vi "Dashboard Main.vi"() -> ()   [LabVIEW 2018]
uses:
  <vilib>/Utility/miscctls.llb/LVRowAndColumnTypeDef.ctl
  <vilib>/event_ctls.llb/eventvkey.ctl
  <vilib>/Rock Robotics/Network Tables/NT Read Numeric Array.vi
  <vilib>/Rock Robotics/Network Tables/NT Write Boolean.vi
  <vilib>/Rock Robotics/Network Tables/NT Read Boolean.vi
  <vilib>/Rock Robotics/WPI/Dashboard/WPI_DashboardLogging Global.vi
panel:
  in  "Camera Settings Right":T1={"Frame Rate"=30, "Compression"=30, "Size"=1, "DB Camera Config"=FALSE} {"Frame Rate" scale=1.0..30.0; "Compression" scale=100.0..-1.0; "Size" items=["640x480", "320x240", "160x120"]}
  in  "Camera Name Right":string(combo)="No Camera Selection"
  out "Camera Perf":string
  in  "Camera Settings":T1={"Frame Rate"=30, "Compression"=30, "Size"=1, "DB Camera Config"=FALSE} {"Frame Rate" scale=1.0..30.0; "Compression" scale=100.0..-1.0; "Size" items=["640x480", "320x240", "160x120"]}
  in  "TCP":refnum<k5>
  in  "Rec Mode":enum32{"Stop", "Record", "Playback"}(radio)
  out "Robot IP":string
  out "Image Message":string="Timeout in Camera Communications"
  in  "Dashboard Tab":T2(tab)
  in  "Select Auto":string(combo)="Select Autonomous ..."
  out "NT Connection":bool
  out "MotorChart R":cluster{"Numeric":dbl, "Numeric":dbl}(graph)
  out "MotorChart L":cluster{"Numeric":dbl, "Numeric":dbl}(graph)
  out "MotorSliders R":cluster{"MotorSlide1":dbl, "MotorSlide2":dbl} {"MotorSlide2" scale=-1.0..1.0 scale format="%#_2e"; "MotorSlide1" scale=-1.0..1.0 scale format="%#_2e"}
  out "MotorSliders L":cluster{"MotorSlide1":dbl, "MotorSlide2":dbl} {"MotorSlide2" scale=-1.0..1.0 scale format="%#_2e"; "MotorSlide1" scale=-1.0..1.0 scale format="%#_2e"}
  out "Gyro":dbl(knob) scale=0.0..360.0
  out "JS1 Z":dbl(slide) scale=-1.0..1.0 scale format="%#_2e"
  out "JS1 Graph":cluster{"X":dbl, "Y":dbl}[](graph)
  out "JS1 Buttons":T3
  out "JS2 Z":dbl(slide) scale=-1.0..1.0 scale format="%#_2e"
  out "JS2 Graph":cluster{"X":dbl, "Y":dbl}[](graph)
  out "JS2 Buttons":T3
  out "Mode":T4(ring)=enum."Auto Disabled"
  out "Right Camera Perf":cluster{"Bandwidth (Mbps)":dbl, "FPS":dbl}
  out "Camera Image Right":T5(plugin-control)
  out "Right Drive Position":dbl
  out "Left Drive Position":dbl
  out "Right Drive Velocity":dbl
  out "Left Drive Velocity":dbl
  out "Hab 3 Triggered":bool
  out "Hatch Device Extended":bool
  out "Gyro 2":dbl(knob) scale=0.0..360.0
  out "Arm Orientation":string
  out "Arm Setpoint":string
  out "Elevator Setpoint":string
  in  "Part Two?":bool
  in  "Start Zone":string(combo)="1"
  in  "Start Position":string(combo)="left"
  in  "Autonomous Selection":string(combo)="0"
  in  "Test Slider":dbl(slide) scale=0.0..100.0 scale format="%#_3g"
  in  "On/Off":bool caption="Solenoid"
  in  "Test Name":u16(ring) items=["Select the test to run..."]
  in  "Test Tree":string(tree)
  in  "Motor":cluster{"Value":dbl, "Enable":bool} {"Value" scale=-1.0..1.0 scale format="%#_3g"}
  out "Progress":T6 {"Test Progress" scale=0.0..100.0}
  in  "Rev/Fwd":cluster{"Forward":bool, "Reverse":bool}
  in  "Test Ring":u16(ring) items=["Monochrome", "Color"]
  out "Cmd Status":string
  in  "Execute Command":bool
  in  "Command Params":string[][](table)
  in  "Command Selection":i32(listbox)
  in  "CheckList":i32(listbox)
  out "Tree":string(tree)
  out "Camera Image":T5(plugin-control)
  out "Background":bool
  in  "Camera Name":string(combo)="No Camera Selection"
  # "HW"
  # "HW"
  # "Joysticks"
  # "Drive Motors"
  # "Front"
  # "Left"
  # "Right"
  # "Back"
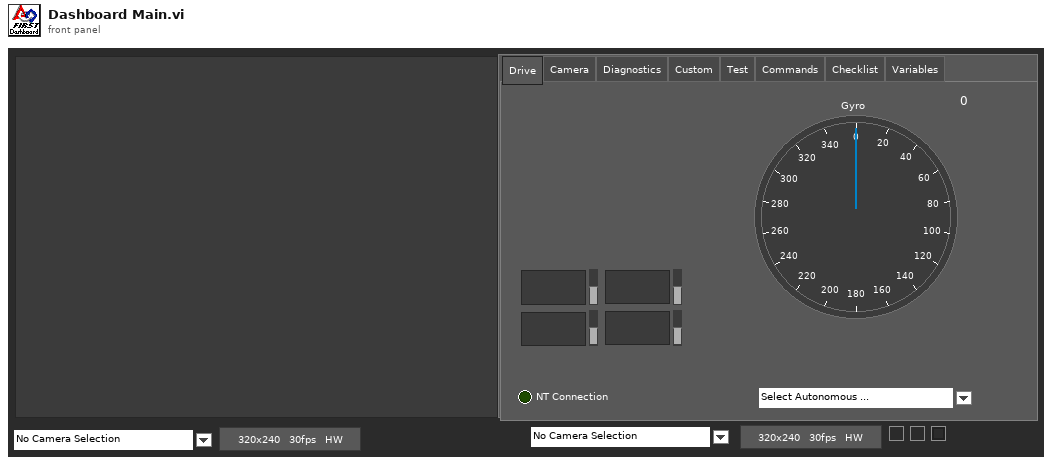
[diagram p1: front panel]
types:
  T1 = cluster{"Frame Rate":i32, "Compression":i32, "Size":u16, "DB Camera Config":bool}
  T2 = enum32{"Drive", "Camera", "Diagnostics", "Custom", "Test", "Commands", "Checklist", "Variables"}
  T3 = cluster{bool, bool, bool, bool, bool, bool, bool, bool, bool, bool, bool, bool}
  T4 = enum8{"Tele-Op Disabled", "Tele-Op Enabled", "Auto Disabled", "Auto Enabled", "Test Disabled", "Test Enabled", "Disconnected", "No Code", "E-Stop"}
  T5 = typedef "IMAQ Image.ctl" = refnum<image>
  T6 = cluster{"Test Progress":u8, "Test Progress Text":string}
  T7 = cluster{"Save Path":path, "Interval (s)":dbl, "Keep":i32}
  T8 = enum32{"Drive", "Camera", "Basic", "Custom", "Test", "Commands", "Checklist", "Variables"}
  T9 = typedef "Image Type" = u32
  T10 = cluster{"IDs":cluster{"RPC field ID":u16, "Unique ID":u16}, "String":string}
  T11 = cluster{"Error Strings":string, "Disable Counts":cluster{u16, u16}, "Rail Faults":cluster{u16, u16, u16}, "Robot IP":string, "DB Mode":u8, "Event Info":cluster{"Name":string, "Type":u8, "Number":u16, "Replay":u8}}
  T12 = cluster{"Storage":cluster{"Disk Free":u64, "RAM Block":u32, "RAM free":u32}, "CPU Utilization":cluster{"CPU % ISR":sgl, "CPU % Time Crit":sgl, "CPU % Timed Str":sgl, "CPU % High":sgl, "CPU % Above":sgl, "CPU % Normal":sgl, "CPU % Low":sgl}, "CAN":cluster{"% Bus Utilization":sgl, "Bus Off Cnt":u32, "TX_FIFO Full Cnt":u32, "Receive Error Cnt":u8, "Transmit Error Cnt":u8}, "HID":cluster{"HID Outputs":u32, "Rumble Low":u16, "Rumble High":u16}[]}
  T13 = cluster{"Status bits":cluster{"Test Mode":bool, "Autonomous":bool, "Enabled":bool, "Code Start":bool, "Brownout":bool, "Reserved 2":bool, "Reserved 3":bool, "E-Stop":bool}, "Code Trace":cluster{"Disabled":bool, "TeleOp":bool, "Auto":bool, "Test":bool}, "Controller Type":enum16{"unknown", "cRIO", "roboRio"}, "Code?":enum16{"unknown", "noCode", "code"}, "Battery V":dbl}
  T14 = cluster{"Control Bits":cluster{"TestMode":bool, "Autonomous":bool, "Enabled":bool, "FMS Present":bool, bool, bool, bool, "E-Stop":bool}, "Team Station ":u8, "Countdown":sgl, "Joystick Values":cluster{"Axes":dbl[], "Buttons":bool[], "POVs":i16[]}[]}
  T15 = cluster{"Axes":dbl[], "Buttons":bool[], "POVs":i16[]}[]
  T16 = cluster{"Axes":dbl[], "Buttons":bool[], "POVs":i16[]}
  T17 = cluster{"Buttons[0]":bool, "Buttons[1]":bool, "Buttons[2]":bool, "Buttons[3]":bool, "Buttons[4]":bool, "Buttons[5]":bool, "Buttons[6]":bool, "Buttons[7]":bool, "Buttons[8]":bool, "Buttons[9]":bool, "Buttons[10]":bool, "Buttons[11]":bool}
  T18 = cluster{"Camera Image":refnum<vi>, "Dashboard Tab":refnum<vi>, "Background":refnum<vi>, "Rec Mode":refnum<vi>, "Test Slider":refnum<vi>, "On/Off ":refnum<vi>, "Test Ring":refnum<vi>, "Rev/Fwd":refnum<vi>, "Test Name":refnum<vi>, "Motor":refnum<vi>, "Progress":refnum<vi>, "CheckList":refnum<vi>, "Tree":refnum<vi>, "Test Tree":refnum<vi>, "Command Params":refnum<vi>, "Command Selection":refnum<vi>, "Execute Command":refnum<vi>, "Cmd Status":refnum<vi>, "Camera Settings":refnum<vi>, "Camera Name":refnum<vi>, "Camera Perf":refnum<vi>, "Camera Settings Right":refnum<vi>, "Camera Name Right":refnum<vi>, "Camera Image Right":refnum<vi>}
  T19 = cluster{"Global Rectangle":i32[], "Contours":cluster{"Contour Type":u32, "ROI Type":u32, "Points":i32[]}[]}
  T20 = cluster{"Camera Name":string, string, "Saved DB Images Info":cluster{"Save Path":path, "Interval (s)":dbl, "Keep":i32}}
  T21 = cluster{"Camera Name Right":string, string, "Saved DB Images Info":cluster{"Save Path":path, "Interval (s)":dbl, "Keep":i32}}
  T22 = cluster{"Operation":enum16{"Update", "Clear"}, "Color Box":u32}[]
  T23 = typedef "eventvkey.ctl" = enum16{"ASCII", "Enter", "Return", "Shift", "Ctrl", "Alt", "Cmd", "Opt", "Caps", "NumLock", "Clear", "Break", "Up", "Down", "Left", "Right", "Insert", "Delete", "Home", "End", "PageUp", "PageDown", "Escape", "Help", "Pause", "ScrollLock", "F1", "F2", "F3", "F4", "F5", "F6", "F7", "F8", "F9", "F10", "F11", "F12", "F13", "F14", "F15", "F16", "F17", "F18", "F19", "F20", "F21", "F22", "F23", "F24", "Play", "VolumeUp", "VolumeDown", "Mute", "Two Byte Char"}
  T24 = cluster{"Image Size":bool, "Image Type":bool, "Pixel Value":bool, "ROI Information":bool, "Zoom Factor":bool}
  T25 = cluster{"Operation":enum16{"Update", "Clear"}, "Color Box":u32}
  T26 = typedef "LVRowAndColumnTypeDef.ctl" = cluster{"Row":i32, "Column":i32}
  T27 = cluster{"Shift":bool, "Ctrl":bool, "Alt":bool, "Cmd":bool, "Opt":bool}
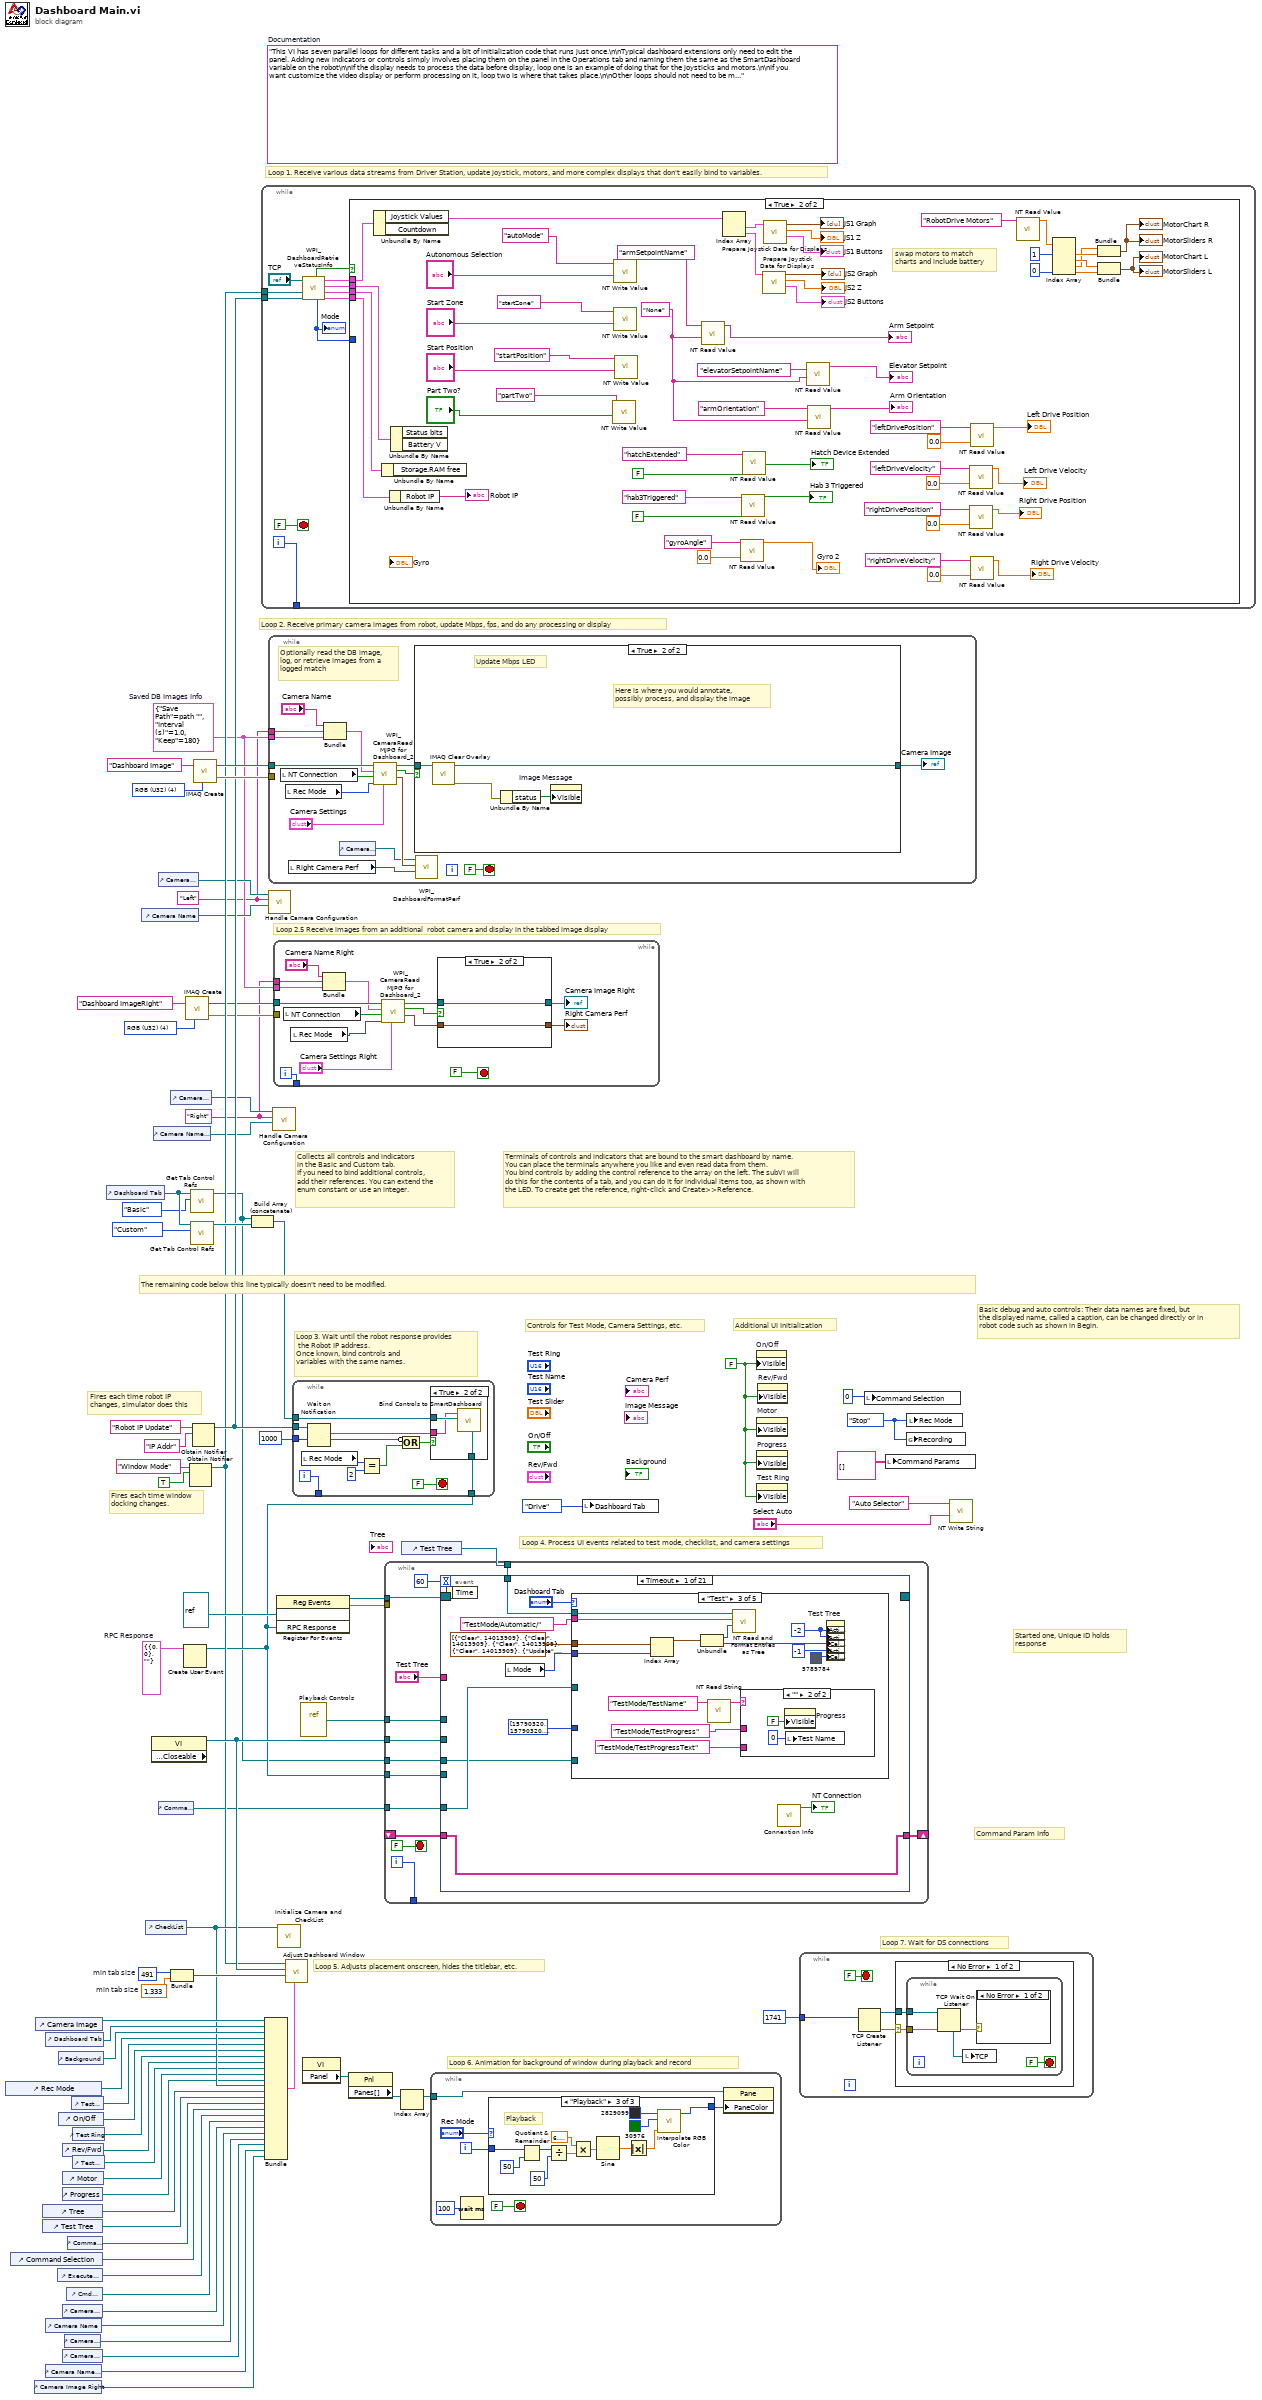
[diagram p0: block diagram]
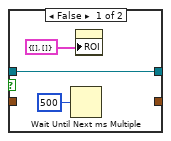
[diagram p2: hidden frame]
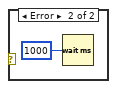
[diagram p3: hidden frame]
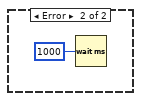
[diagram p4: hidden frame]
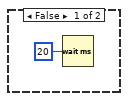
[diagram p5: hidden frame]
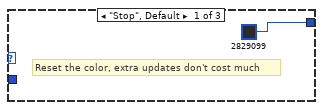
[diagram p6: hidden frame]
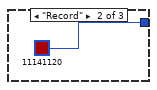
[diagram p7: hidden frame]
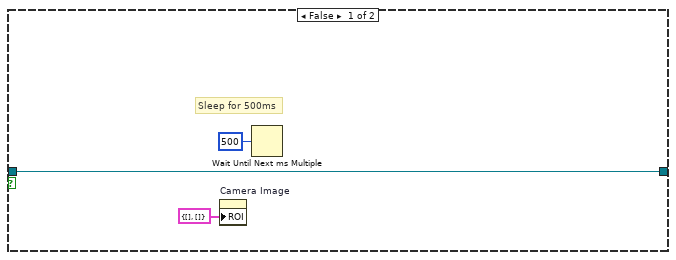
[diagram p9: hidden frame]
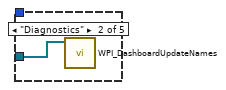
[diagram p11: hidden frame]
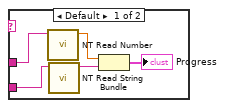
[diagram p12: hidden frame]
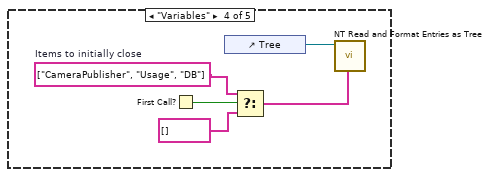
[diagram p13: hidden frame]
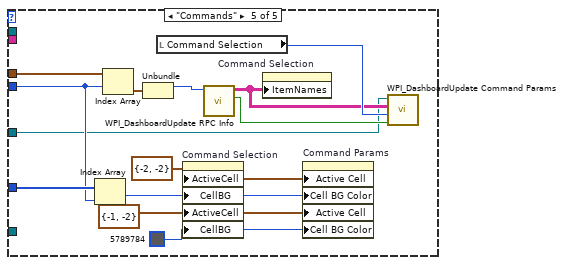
[diagram p14: hidden frame]
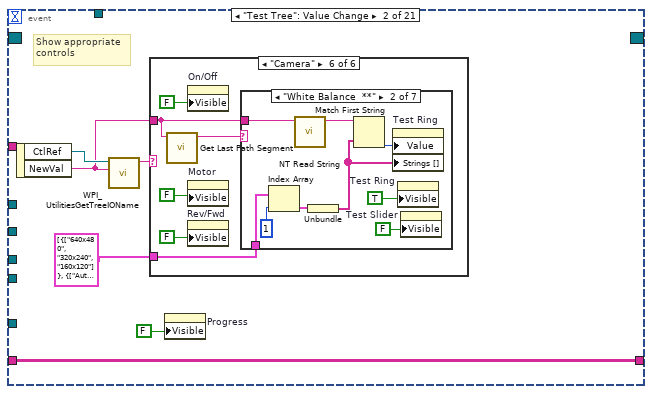
[diagram p15: hidden frame]
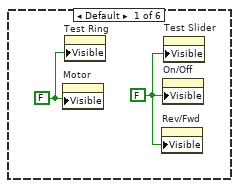
[diagram p16: hidden frame]
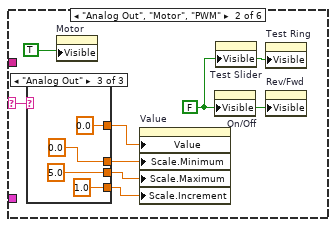
[diagram p17: hidden frame]
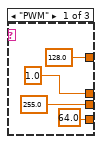
[diagram p18: hidden frame]
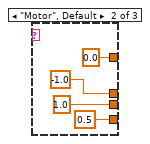
[diagram p19: hidden frame]
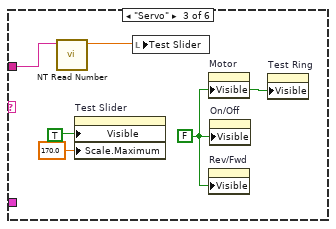
[diagram p20: hidden frame]
diagram:
  w4 = T7 {"Save Path"=path "", "Interval (s)"=1.0, "Keep"=180}  # Saved DB Images Info
  w3 = "Right"
  w2 = "Left"
  w14 = T9 4 items=["Grayscale (U8)", "Grayscale (I16)", "Grayscale (SGL)", "Complex (CSG)", "RGB (U32)", "HSL (U32)", "RGB (U64)"] ("Image Type")
  w30 = T10 {"IDs"={"RPC field ID"=0, "Unique ID"=0}, "String"=""}  # RPC Response
  w52 = 491  # min tab size
  w51 = 1.333  # min tab size
  w59 = enum32{"Stop", "Record", "Playback"}."Stop" ("Rec Mode")
  w36 = FALSE ("Visible")
  (unwired) "This VI has seven parallel loops for different tasks and a bit of initialization code that runs just once.\n\nTypical dashboard extensions only need to edit the panel. Adding new indicators or controls simply involves placing them on the panel in the Operations tab and naming them the same as the SmartDashboard variable on the robot\n\nIf the display needs to process the data before display, loop one is an example of doing that for the joysticks and motors.\n\nIf you want customize the video display or perform processing on it, loop two is where that takes place.\n\nOther loops should not need to be modified. They are pretty standard, and document the task they perform."  # Documentation
  w76 = T9 4 items=["Grayscale (U8)", "Grayscale (I16)", "Grayscale (SGL)", "Complex (CSG)", "RGB (U32)", "HSL (U32)", "RGB (U64)"] ("Image Type")
  # "Loop 2.5 Receive images from an additional  robot camera and display in the tabbed image display"
  # "Command Param Info"
  # "Started one, Unique ID holds\nresponse"
  # "Loop 7. Wait for DS connections"
  # "Basic debug and auto controls: Their data names are fixed, but\nthe displayed name, called a caption, can be changed directly or in\nrobot code such as shown in Begin."
  # "Controls for Test Mode, Camera Settings, etc."
  # "Additional UI Initialization"
  # "Loop 6. Animation for background of window during playback and record"
  # "Fires each time robot IP\nchanges, simulator does this"
  # "Fires each time window\ndocking changes."
  # "Collects all controls and indicators\nin the Basic and Custom tab.\nIf you need to bind additional controls,\nadd their references. You can extend the\nenum constant or use an integer."
  # "The remaining code below this line typically doesn't need to be modified."
  # "Loop 4. Process UI events related to test mode, checklist, and camera settings"
  # "Terminals of controls and indicators that are bound to the smart dashboard by name.\nYou can place the terminals anywhere you like and even read data from them.\nYou bind controls by adding the control reference to the array on the left. The subVI will\ndo this for the contents of a tab, and you can do it for individual items too, as shown with\nthe LED. To create get the reference, right-click and Create>>Reference."
  # "Loop 3. Wait until the robot response provides\n the Robot IP address.\nOnce known, bind controls and\nvariables with the same names."
  # "Loop 5. Adjusts placement onscreen, hides the titlebar, etc."
  # "Loop 1. Receive various data streams from Driver Station, update joystick, motors, and more complex displays that don't easily bind to variables."
  # "Loop 2. Receive primary camera images from robot, update Mbps, fps, and do any processing or display"
  n1 = control-ref of="Rec Mode"() -> (w42:refnum<vi>)
  n2 = control-ref of="Command Selection"() -> (w29:refnum<vi>)
  n3 = control-ref of="Camera Image Right"() -> (w7:refnum<vi>)
  n4 = control-ref of="Camera Image"() -> (w54:refnum<vi>)
  n5 = control-ref of="Tree"() -> (w46:refnum<vi>)
  n6 = control-ref of="Test Tree"() -> (w45:refnum<vi>)
  n7 = control-ref of="Dashboard Tab"() -> (w53:refnum<vi>)
  n8 = control-ref of="Camera Name"() -> (w20:refnum<vi>)
  n9 = control-ref of="Camera Name Right"() -> (w8:refnum<vi>)
  n10 = control-ref of="Execute Command"() -> (w31:refnum<vi>)
  n11 = control-ref of="Background"() -> (w49:refnum<vi>)
  n12 = control-ref of="On/Off"() -> (w40:refnum<vi>)
  n13 = control-ref of="Progress"() -> (w37:refnum<vi>)
  n14 = control-ref of="Camera Settings"() -> (w21:refnum<vi>)
  n15 = control-ref of="Camera Settings Right"() -> (w9:refnum<vi>)
  n16 = control-ref of="Rev/Fwd"() -> (w38:refnum<vi>)
  n17 = control-ref of="Motor"() -> (w43:refnum<vi>)
  n18 = control-ref of="Camera Perf"() -> (w19:refnum<vi>)
  n19 = control-ref of="Cmd Status"() -> (w25:refnum<vi>)
  n20 = control-ref of="Command Params"() -> (w32:refnum<vi>)
  n21 = control-ref of="Test Slider"() -> (w41:refnum<vi>)
  n22 = control-ref of="Test Ring"() -> (w39:refnum<vi>)
  n23 = control-ref of="Test Name"() -> (w44:refnum<vi>)
  n24 = control-ref of="Dashboard Tab"() -> (w57:refnum<vi>)
  n25 = control-ref of="Camera Name"() -> (w22:refnum<vi>)
  n26 = control-ref of="CheckList"() -> (w47:refnum<vi>)
  n27 = property class="VI" props=["Front Panel.Closeable"]() -> (reference out=w58:refnum<vi>)  [unwired: 2 in, 2 out]
  n28 = control-ref of="Camera Name Right"() -> (w10:refnum<vi>)
  n29 = control-ref of="Camera Settings"() -> (w23:refnum<vi>)
  n30 = control-ref of="Command Params"() -> (w24:refnum<vi>)
  n31 = control-ref of="Camera Settings Right"() -> (w11:refnum<vi>)
  n32 = Bundle("min tab size"=w52, "min tab size"=w51) -> (w50:cluster{"min tab size":i32, "min tab size":dbl})  [unwired: 1 in]
  n33 = Create User Event(user event datatype=w30) -> (user event=w26:refnum<user-event>)  [unwired: 1 in, 1 out]
  n34 = call "IMAQ Create"("Image Name"="Dashboard ImageRight", "Image Type"=w14) -> ("New Image"=w13:T5, "error out"=w12:errorcluster)  [unwired: 2 in, 1 out]
  n35 = Obtain Notifier(name (unnamed)="Window Mode", notification data type=TRUE) -> (notifier out=w34:refnum<notifier>)  [unwired: 2 in, 2 out]
  n36 = call <vilib>:"Get Tab Control Refs.vi"("Page Index"=T8."Basic" ("Dashboard Tab"), "TabControl in"=w57) -> ("ControlsOnPage"=w18:refnum<vi>[])  [unwired: 9 in]
  n37 = call <vilib>:"Get Tab Control Refs.vi"("Page Index"=T8."Custom" ("Dashboard Tab"), "TabControl in"=w57) -> ("ControlsOnPage"=w56:refnum<vi>[])  [unwired: 9 in]
  n38 = Obtain Notifier(name (unnamed)="Robot IP Update", notification data type="IP Addr" ("name (unnamed)")) -> (notifier out=w35:refnum<notifier>)  [unwired: 2 in, 2 out]
  n39 = call "IMAQ Create"("Image Name"="Dashboard Image", "Image Type"=w76) -> ("New Image"=w74:T5, "error out"=w73:errorcluster)  [unwired: 2 in, 1 out]
  n40 = Build Array (concatenate)(w18, w56) -> (w55:refnum<vi>[])
  n41 = while {
    tunnel: [w86] -> _
    tunnel: w35 -> [w80]
    tunnel: w34 -> [w77]
    i -> [w86]
    stop <- FALSE stop-if-true
    n42 = call <vilib>:"WPI_DashboardRetrieveStatusInfo.vi"("Binding Refnum"=w80, "Window Mode Notifier"=w77, "TCP Cnx"="TCP") -> ("Power and Errors"=w81:T11, "Robot Metrics"=w84:T12, "Status Info"=w85:T13, "Control Info"=w82:T14, "Robot Mode"=w79:T4, "Process?"=w83:bool)  [unwired: 3 in]
    "Mode" <- w79
    n43 = case shown="True" w83 {
      tunnel: w85 -> [_ w148]
      tunnel: w84 -> [_ w147]
      tunnel: w82 -> [_ w146]
      tunnel: w81 -> [_ w145]
      tunnel: w79 -> [_ _]
      frame False {
        n44 = Wait (ms)(milliseconds to wait=u32 20) -> ()  [unwired: 1 out]
      }
      frame True {
        w110 = "None" ("Default Value")
        # "swap motors to match\ncharts and include battery"
        n45 = Unbundle By Name(w146) -> ("Joystick Values"=w136:T15)  [unwired: 1 out]
        n46 = Unbundle By Name(w147) -> ()  [unwired: 1 out]
        n47 = Unbundle By Name(w145) -> ("Robot IP"=→"Robot IP":string)
        n48 = Unbundle By Name(w148) -> ()  [unwired: 2 out]
        n49 = call-poly <vilib>:"NT Write Value.vi"("Boolean"="Part Two?", "Name"="partTwo") -> ()  [unwired: 9 in, 1 out]
        n50 = call-poly <vilib>:"NT Write Value.vi"("String"="Autonomous Selection", "Name"="autoMode") -> ()  [unwired: 9 in, 1 out]
        n51 = call-poly <vilib>:"NT Write Value.vi"("String"="Start Zone", "Name"="startZone") -> ()  [unwired: 9 in, 1 out]
        n52 = call-poly <vilib>:"NT Write Value.vi"("String"="Start Position", "Name"="startPosition") -> ()  [unwired: 9 in, 1 out]
        n53 = call-poly <vilib>:"NT Read Value.vi"("Default Value"=w110, "Name"="armSetpointName") -> ("String"=→"Arm Setpoint":string)  [unwired: 8 in, 1 out]
        n54 = Index Array(array=w136) -> (element #1=w135:T16, element #2=w131:T16)  [unwired: 2 in]
        n55 = call-poly <vilib>:"NT Read Value.vi"("Default Value"=0.0, "Name"="gyroAngle") -> ("Numeric"=→"Gyro 2":dbl)  [unwired: 8 in, 1 out]
        n56 = call-poly <vilib>:"NT Read Value.vi"("Default Value"=FALSE, "Name"="hab3Triggered") -> ("Boolean"=→"Hab 3 Triggered":bool)  [unwired: 8 in, 1 out]
        n57 = call-poly <vilib>:"NT Read Value.vi"("Default Value"=FALSE, "Name"="hatchExtended") -> ("Boolean"=→"Hatch Device Extended":bool)  [unwired: 8 in, 1 out]
        n58 = call "Prepare Joystick Data for Displays.vi"("Joystick Values"=w131) -> ("Buttons"=→"JS2 Buttons":T17, "Z Axis"=→"JS2 Z":dbl, "Cartesian Data"=→"JS2 Graph":cluster{"X axis":dbl, "X axis":dbl}[])  [unwired: 8 in]
        n59 = call "Prepare Joystick Data for Displays.vi"("Joystick Values"=w135) -> ("Buttons"=→"JS1 Buttons":T17, "Z Axis"=→"JS1 Z":dbl, "Cartesian Data"=→"JS1 Graph":cluster{"X axis":dbl, "X axis":dbl}[])  [unwired: 8 in]
        n60 = call-poly <vilib>:"NT Read Value.vi"("Default Value"=w110, "Name"="elevatorSetpointName") -> ("String"=→"Elevator Setpoint":string)  [unwired: 8 in, 1 out]
        n61 = call-poly <vilib>:"NT Read Value.vi"("Default Value"=w110, "Name"="armOrientation") -> ("String"=→"Arm Orientation":string)  [unwired: 8 in, 1 out]
        n62 = call-poly <vilib>:"NT Read Value.vi"("Default Value"=0.0, "Name"="leftDriveVelocity") -> ("Numeric"=→"Left Drive Velocity":dbl)  [unwired: 8 in, 1 out]
        n63 = call-poly <vilib>:"NT Read Value.vi"("Default Value"=0.0, "Name"="rightDrivePosition") -> ("Numeric"=→"Right Drive Position":dbl)  [unwired: 8 in, 1 out]
        n64 = call-poly <vilib>:"NT Read Value.vi"("Default Value"=0.0, "Name"="leftDrivePosition") -> ("Numeric"=→"Left Drive Position":dbl)  [unwired: 8 in, 1 out]
        n65 = call-poly <vilib>:"NT Read Value.vi"("Default Value"=0.0, "Name"="rightDriveVelocity") -> ("Numeric"=→"Right Drive Velocity":dbl)  [unwired: 8 in, 1 out]
        n66 = call-poly <vilib>:"NT Read Value.vi"("Name"="RobotDrive Motors") -> ("Numeric Array"=w126:dbl[])  [unwired: 9 in, 1 out]
        n67 = Index Array(array=w126, index #1=1, index #4=0) -> (element #1=w140:dbl, element #2=w141:dbl, element #3=w139:dbl, element #4=w144:dbl)  [unwired: 2 in]
        n68 = Bundle("Numeric"=w139, "Numeric"=w140) -> (→"MotorChart R" →"MotorSliders R":cluster{"Numeric":dbl, "Numeric":dbl})  [unwired: 1 in]
        n69 = Bundle("Numeric"=w141, "Numeric"=w144) -> (→"MotorChart L" →"MotorSliders L":cluster{"Numeric":dbl, "Numeric":dbl})  [unwired: 1 in]
      }
    }
  }
  n70 = Bundle("Camera Image"=w54, "Dashboard Tab"=w53, "Background"=w49, "Rec Mode"=w42, "Test Slider"=w41, "On/Off"=w40, "Test Ring"=w39, "Rev/Fwd"=w38, "Test Name"=w44, "Motor"=w43, "Progress"=w37, "CheckList"=w47, "Tree"=w46, "Test Tree"=w45, "Command Params"=w32, "Command Selection"=w29, "Execute Command"=w31, "Cmd Status"=w25, "Camera Settings"=w21, "Camera Name"=w20, "Camera Perf"=w19, "Camera Settings Right"=w9, "Camera Name Right"=w8, "Camera Image Right"=w7) -> (w48:T18)  [unwired: 1 in]
  n71 = call "Handle Camera Configuration.vi"("CameraNameRef"=w22, "Display Name"=w2, "ClusterRef"=w23) -> ()  [unwired: 9 in]
  n72 = while {
    tunnel: w74 -> [w162]
    tunnel: w73 -> [_]
    tunnel: w4 -> [w155]
    tunnel: w2 -> [w152]
    stop <- FALSE stop-if-true
    # "Optionally read the DB image,\nlog, or retrieve images from a\nlogged match"
    n73 = local read "NT Connection"() -> (w156:bool)
    n74 = local read "Rec Mode"() -> (w159:enum32{"Stop", "Record", "Playback"})
    n75 = local read "Right Camera Perf"() -> (w150:cluster{"Bandwidth (Mbps)":dbl, "FPS":dbl})
    n76 = Bundle("Camera Name"="Camera Name", w152, "Saved DB Images Info"=w155) -> (w154:T20)  [unwired: 1 in]
    n77 = control-ref of="Camera Perf"() -> (w149:refnum<vi>)
    n78 = call <vilib>:"WPI_CameraRead MJPG for Dashboard_2.vi"("Camera Settings"="Camera Settings", "Rec Mode"=w159, "NT Connection"=w156, "Capture Info"=w154, "Image in"=w162) -> ("perf info"=w151:cluster{"Bandwidth (Mbps)":dbl, "fps":dbl}, "Active"=w160:bool, "Image\\ out"=w161:T5)  [unwired: 4 in]
    n79 = case shown="True" w160 {
      tunnel: w161 -> [w165 w168]
      tunnel: [w165 w167] -> w157
      frame False {
        # "Sleep for 500ms"
        n80 = property on="Camera Image" class="ImageControl"("ROI"=T19 {"Global Rectangle"=[], "Contours"=[]}) -> ()  [unwired: 2 in, 2 out]
        n81 = Wait Until Next ms Multiple(millisecond multiple=u32 500) -> ()  [unwired: 1 out]
      }
      frame True {
        # "Here is where you would annotate,\npossibly process, and display the image"
        # "Update Mbps LED"
        n82 = call "IMAQ Clear Overlay"("Image"=w168) -> ("error out"=w169:errorcluster, "Image Out"=w167:T5)  [unwired: 2 in, 7 out]
        n83 = Unbundle By Name(w169) -> ("status"=w170:bool)
        n84 = property on="Image Message" class="Str"("Visible"=w170) -> ()  [unwired: 2 in, 2 out]
      }
    }
    "Camera Image" <- w157
    n85 = call <vilib>:"WPI_DashboardFormatPerf.vi"("Right Camera Perf"=w150, "Performance"=w151, "String in"=w149) -> ()  [unwired: 9 in]
  }
  n86 = call "Handle Camera Configuration.vi"("CameraNameRef"=w10, "Display Name"=w3, "ClusterRef"=w11) -> ()  [unwired: 9 in]
  n87 = while {
    tunnel: w13 -> [w185]
    tunnel: w12 -> [_]
    tunnel: [w180] -> _
    tunnel: w4 -> [w176]
    tunnel: w3 -> [w173]
    i -> [w180]
    stop <- FALSE stop-if-true
    n88 = local read "NT Connection"() -> (w177:bool)
    n89 = local read "Rec Mode"() -> (w184:enum32{"Stop", "Record", "Playback"})
    n90 = Bundle("Camera Name Right"="Camera Name Right", w173, "Saved DB Images Info"=w176) -> (w175:T21)  [unwired: 1 in]
    n91 = call <vilib>:"WPI_CameraRead MJPG for Dashboard_2.vi"("Camera Settings"="Camera Settings Right", "Rec Mode"=w184, "NT Connection"=w177, "Capture Info"=w175, "Image in"=w185) -> ("perf info"=w171:cluster{"Bandwidth (Mbps)":dbl, "fps":dbl}, "Active"=w179:bool, "Image\\ out"=w182:T5)  [unwired: 4 in]
    n92 = case shown="True" w179 {
      tunnel: w182 -> [w187 w190]
      tunnel: [w187 w190] -> w178
      tunnel: [_ w189] -> w172
      tunnel: w171 -> [_ w189]
      frame False {
        n93 = Wait Until Next ms Multiple(millisecond multiple=u32 500) -> ()  [unwired: 1 out]
        n94 = property on="Camera Image Right" class="ImageControl"("ROI"=T19 {"Global Rectangle"=[], "Contours"=[]}) -> ()  [unwired: 2 in, 2 out]
      }
      frame True {
      }
    }
    "Camera Image Right" <- w178
    "Right Camera Perf" <- w172
  }
  n95 = register-events(refnum<vi> refnum, w26) -> (reference out=w63:refnum<event-registration>, error out=w62:errorcluster)  [unwired: 2 in]
  n96 = call "Initialize Camera and CheckList.vi"("ListBox in"=w47) -> ()  [unwired: 11 in]
  n97 = call "Adjust Dashboard Window.vi"("Sizing Refnums"=w48, "Size Constraints"=w50, "VI"=w58, "WIn Mode"=w34) -> ()  [unwired: 8 in]
  n98 = while {
    tunnel: w55 -> [w202]
    tunnel: w35 -> [w200]
    tunnel: [w198] -> _
    tunnel: u32 1000 ("milliseconds to wait") -> [w197]
    tunnel: w26 -> [w191]
    i -> [w198]
    stop <- FALSE stop-if-true
    n99 = local read "Rec Mode"() -> (w193:enum32{"Stop", "Record", "Playback"})
    n100 = Wait on Notification(notifier=w200, timeout in ms (-1)=w197) -> (notification=w199:string, timed out?=w195:bool)  [unwired: 2 in, 2 out]
    n101 = Equal?(x=w193, y=u16 2 ("Rec Mode")) -> (x = y?=w194:bool)
    n102 = Compound Arithmetic op=OR(invert w195, w194) -> (w196:bool)
    n103 = case shown="True" w196 {
      tunnel: w202 -> [_ w205]
      tunnel: w199 -> [_ w204]
      tunnel: w191 -> [_ w203]
      frame False {
      }
      frame True {
        n104 = call <vilib>:"Bind Controls to SmartDashboard.vi"("RPC ref"=w203, "Bound Control Refs"=w205, "Server IP Address"=w204) -> ()  [unwired: 9 in]
      }
    }
  }
  n105 = vi-ref "Playback Controls.vi"() -> (w64:refnum<vi>)
  n106 = property class="VI"() -> ("Panel"=w66:refnum<vi>)  [unwired: 2 in, 2 out]
  n107 = property class="Pnl"(reference=w66) -> ("Panes[]"=w67:refnum<vi>[])  [unwired: 1 in, 2 out]
  n108 = Index Array(array=w67) -> (element=w65:refnum<vi>)  [unwired: 1 in]
  n109 = control-ref of="Test Tree"() -> (w68:refnum<vi>)
  n110 = while {
    tunnel: [w215] -> _
    tunnel: w68 -> [w214]
    tunnel: w64 -> [w213]
    tunnel: w63 -> [w212]
    tunnel: w62 -> [_]
    tunnel: w58 -> [w211]
    tunnel: w26 -> [w210]
    tunnel: w24 -> [w209]
    shift-right: [w208] -> _
    shift-left: _ -> [w207]
    tunnel: w18 -> [w206]
    i -> [w215]
    stop <- FALSE stop-if-true
    n111 = event shown="[0] Timeout" {
      selector: w212 -> [_ _ _ _ _ _ _ _ _ _ _ _ _ _ _ _ _ _ _ _ _]
      dyn-events: [_ _ _ _ _ _ _ _ _ _ _ _ _ _ _ _ w475 _ _ _ _] -> _
      timeout: u32 60 ("milliseconds to wait") -> [_ _ _ _ _ _ _ _ _ _ _ _ _ _ _ _ _ _ _ _ _]
      tunnel: w214 -> [w227 _ _ _ _ _ _ _ _ _ _ _ _ _ _ _ _ _ _ _ _]
      tunnel: "Test Tree" -> [_ _ _ _ _ _ _ _ _ _ _ w442 w450 w452 w456 w464 _ _ _ _ _]
      tunnel: w213 -> [_ _ _ _ _ _ _ _ _ _ _ _ _ _ _ _ w477 _ w495 _ _]
      tunnel: w211 -> [_ _ _ _ _ _ _ _ _ _ _ _ _ _ _ _ w473 _ _ _ _]
      tunnel: w210 -> [_ _ _ _ _ _ _ _ _ _ _ _ _ _ _ _ w471 _ _ _ _]
      tunnel: w209 -> [w222 _ _ _ _ _ w393 _ _ _ _ _ _ _ _ _ _ _ _ _ _]
      tunnel: [w221 w270 w372 w377 w386 w390 w391 w400 w410 w417 w429 w441 w448 w451 w455 w463 w470 w490 w492 w496 w509] -> w208
      tunnel: w207 -> [w221 w270 w372 w377 w386 w390 w391 _ _ w417 w429 w441 w448 w451 w455 w463 w470 w490 w492 w496 w509]
      tunnel: w206 -> [w219 _ _ _ _ _ _ _ _ _ _ _ _ _ _ _ _ _ _ _ _]
      event Timeout {
        n112 = event-data() -> ()  [unwired: 1 in, 1 out]
        n113 = local read "Mode"() -> (w224:T4)
        n114 = case shown="\"Test\"" "Dashboard Tab" {
          tunnel: w227 -> [_ _ w243 _ _]
          tunnel: "TestMode/Automatic/" ("Name Pattern") -> [_ _ w242 _ _]
          tunnel: T22 [{"Operation"=enum."Clear", "Color Box"=14013909}, {"Operation"=enum."Clear", "Color Box"=14013909}, {"Operation"=enum."Clear", "Color Box"=14013909}, {"Operation"=enum."Clear", "Color Box"=14013909}, {"Operation"=enum."Update", "Color Box"=14013909}, {"Operation"=enum."Update", "Color Box"=16777215}, {"Operation"=enum."Clear", "Color Box"=14013909}, {"Operation"=enum."Clear", "Color Box"=14013909}, {"Operation"=enum."Clear", "Color Box"=14013909}] -> [_ _ w235 _ w263]
          tunnel: w224 -> [_ _ w234 _ w262]
          tunnel: u32[] [15790320, 15790320, 15790320, 15790320, 16777215, 16777215, 15790320, 15790320, 15790320] -> [_ _ _ _ w268]
          tunnel: w222 -> [_ _ _ _ w256]
          tunnel: w219 -> [_ w229 _ _ _]
          frame "Custom", Default {
          }
          frame "Diagnostics" {
            n115 = call <vilib>:"WPI_DashboardUpdateNames.vi"("Controls on Tab"=w229) -> ()  [unwired: 11 in]
          }
          frame "Test" {
            w241 = -2 ("Active Item:Row Number")
            n116 = Index Array(array=w235, index=w234) -> (element=w236:T25)
            n117 = Unbundle(w236) -> ("Operation"=w237:enum16{"Update", "Clear"}, "Color Box"=w238:u32)
            n118 = call <vilib>:"NT Read String.vi"("Name"="TestMode/TestName") -> ("String"=w232:string)  [unwired: 9 in, 1 out]
            n119 = call <vilib>:"NT Read and Format Entries as Tree.vi"("Operation"=w237, "Name Pattern"=w242, "Tree Refnum"=w243) -> ()  [unwired: 7 in, 2 out]
            n120 = case shown="\"\"" w232 {
              tunnel: "TestMode/TestProgress" ("Name") -> [w245 _]
              tunnel: "TestMode/TestProgressText" ("Name") -> [w244 _]
              frame Default {
                n121 = call <vilib>:"NT Read Number.vi"("Name"=w245) -> ("Numeric"=w246:dbl)  [unwired: 9 in, 1 out]
                n122 = call <vilib>:"NT Read String.vi"("Name"=w244) -> ("String"=w247:string)  [unwired: 9 in, 1 out]
                n123 = Bundle("Numeric"=w246, "String"=w247) -> (→"Progress":cluster{"Numeric":dbl, "String":string})  [unwired: 1 in]
              }
              frame "" {
                n124 = property on="Progress" class="Clust (strict)"("Visible"=FALSE) -> ()  [unwired: 2 in, 2 out]
                n125 = local write "Test Name"(u16 0) -> ()
              }
            }
            n126 = property on="Test Tree" class="Tree (strict)"("Active Item Row Number"=w241, "ActiveColNum"=w241, "CellBG"=w238, "Active Item Row Number"=-1 ("Active Item:Row Number"), "CellBG"=u32 5789784 ("Color Box")) -> ()  [unwired: 2 in, 2 out]
          }
          frame "Variables" {
            w253 = string[] ["CameraPublisher", "Usage", "DB"]  # Items to initially close
            n127 = First Call?() -> (First Call?: T/F=w254:bool)
            n128 = control-ref of="Tree"() -> (w255:refnum<vi>)
            n129 = Select(t=w253, s=w254, f=string[] []) -> (s? t:f=w251:string[])
            n130 = call <vilib>:"NT Read and Format Entries as Tree.vi"("Tags to  Close"=w251, "Tree Refnum"=w255) -> ()  [unwired: 8 in, 2 out]
          }
          frame "Commands" {
            w264 = u32 5789784 ("Color Box")
            w265 = T26 {"Row"=-1, "Column"=-2} ("Active Cell:Active Cell")
            w267 = T26 {"Row"=-2, "Column"=-2} ("Active Cell:Active Cell")
            n131 = Index Array(array=w268, index=w262) -> (element=w266:u32)
            n132 = Index Array(array=w263, index=w262) -> (element=w261:T25)
            n133 = Unbundle(w261) -> ("Operation"=w260:enum16{"Update", "Clear"})  [unwired: 1 out]
            n134 = local read "Command Selection"() -> (w259:i32)
            n135 = property on="Command Selection" class="MCListbox (strict)"("ActiveCell"=w267, "CellBG"=w266, "ActiveCell"=w265, "CellBG"=w264) -> ()  [unwired: 2 in, 2 out]
            n136 = call <vilib>:"WPI_DashboardUpdate RPC Info.vi"("Operation"=w260) -> ("update"=w258:bool, "commands"=w257:string[][])  [unwired: 9 in]
            n137 = property on="Command Selection" class="MCListbox (strict)"("ItemNames"=w257) -> ()  [unwired: 2 in, 2 out]
            n138 = property on="Command Params" class="Tbl (strict)"("Active Cell"=w267, "Cell BG Color"=w266, "Active Cell"=w265, "Cell BG Color"=w264) -> ()  [unwired: 2 in, 2 out]
            n139 = call <vilib>:"WPI_DashboardUpdate Command Params.vi"("Update"=w258, "NewVal"=w259, "Commands"=w257, "Param Tbl"=w256) -> ()  [unwired: 7 in, 1 out]
          }
        }
        n140 = call <vilib>:"Connextion Info.vi"() -> ("Connected"=→"NT Connection":bool)  [unwired: 10 in, 1 out]
      }
      event "Test Tree": Value Change {
        # "Show appropriate\ncontrols"
        n141 = event-data() -> ("CtlRef"=w273:refnum<vi>, "NewVal"=w271:string)  [unwired: 1 in]
        n142 = call <vilib>:"WPI_UtilitiesGetTreeIOName.vi"("NewVal"=w271, "TreeControl in"=w273) -> ("I/O Name"=w274:string)  [unwired: 9 in]
        n143 = case shown="\"Camera\"" w274 {
          selector: w274 -> [_ w281 _ w303 w312 _]
          tunnel: w271 -> [_ _ w300 w302 _ w319]
          tunnel: cluster{string[]}[] [{["640x480", "320x240", "160x120"]}, {["Auto", "Fixed indoor", "Fixed outdoor 1", "Fixed outdoor 2", "Fixed fluorescent 1", "Fixed fluorescent 2", "Hold current"]}, {["Auto", "Flicker-free 50 Hz", "Flicker-free 60 Hz", "Hold current"]}, {["None", "Prioritize frame rate", "Prioritize image quality"]}, {["Monochrome", "Color"]}] -> [_ _ _ _ _ w318]
          frame Default {
            w276 = FALSE ("Visible")
            w275 = FALSE ("Visible")
            n144 = property on="Motor" class="Clust (strict)"("Visible"=w275) -> ()  [unwired: 2 in, 2 out]
            n145 = property on="Test Ring" class="Ring (strict)"("Visible"=w275) -> ()  [unwired: 2 in, 2 out]
            n146 = property on="Rev/Fwd" class="Clust (strict)"("Visible"=w276) -> ()  [unwired: 2 in, 2 out]
            n147 = property on="On/Off" class="Bool (strict)"("Visible"=w276) -> ()  [unwired: 2 in, 2 out]
            n148 = property on="Test Slider" class="Slide (strict)"("Visible"=w276) -> ()  [unwired: 2 in, 2 out]
          }
          frame "Analog Out", "Motor", "PWM" {
            w282 = FALSE ("Visible")
            n149 = case shown="\"Analog Out\"" w281 {
              tunnel: [1.0 ("Value") -1.0 ("Value") 0.0 ("Value")] -> w280
              tunnel: [255.0 ("Value") 1.0 ("Value") 5.0 ("Value")] -> w279
              tunnel: [128.0 ("Value") 0.0 ("Value") 0.0 ("Value")] -> w278
              tunnel: [64.0 ("Value") 0.5 ("Value") 1.0 ("Value")] -> w277
              frame "PWM" {
              }
              frame "Motor", Default {
              }
              frame "Analog Out" {
              }
            }
            n150 = property on="Motor" class="Clust (strict)"("Visible"=TRUE) -> ()  [unwired: 2 in, 2 out]
            n151 = property on="Value" class="Slide (strict)"("Value"=w278, "Scale.Minimum"=w280, "Scale.Maximum"=w279, "Scale.Increment"=w277) -> ()  [unwired: 2 in, 2 out]
            n152 = property on="On/Off" class="Bool (strict)"("Visible"=w282) -> ()  [unwired: 2 in, 2 out]
            n153 = property on="Test Slider" class="Slide (strict)"("Visible"=w282) -> ()  [unwired: 2 in, 2 out]
            n154 = property on="Test Ring" class="Ring (strict)"("Visible"=w282) -> ()  [unwired: 2 in, 2 out]
            n155 = property on="Rev/Fwd" class="Clust (strict)"("Visible"=w282) -> ()  [unwired: 2 in, 2 out]
          }
          frame "Servo" {
            w298 = FALSE ("Visible")
            n156 = call <vilib>:"NT Read Number.vi"("Name"=w300) -> ("Numeric"=w299:dbl)  [unwired: 9 in, 1 out]
            n157 = property on="Test Slider" class="Slide (strict)"("Visible"=TRUE, "Scale.Maximum"=170.0 ("Scale.Range:Maximum")) -> ()  [unwired: 2 in, 2 out]
            n158 = local write "Test Slider"(w299) -> ()
            n159 = property on="Motor" class="Clust (strict)"("Visible"=w298) -> ()  [unwired: 2 in, 2 out]
            n160 = property on="Rev/Fwd" class="Clust (strict)"("Visible"=w298) -> ()  [unwired: 2 in, 2 out]
            n161 = property on="On/Off" class="Bool (strict)"("Visible"=w298) -> ()  [unwired: 2 in, 2 out]
            n162 = property on="Test Ring" class="Ring (strict)"("Visible"=w298) -> ()  [unwired: 2 in, 2 out]
          }
          frame "Relay", "Solenoid" {
            w301 = FALSE ("Visible")
            n163 = property on="Motor" class="Clust (strict)"("Visible"=w301) -> ()  [unwired: 2 in, 2 out]
            n164 = property on="Test Slider" class="Slide (strict)"("Visible"=w301) -> ()  [unwired: 2 in, 2 out]
            n165 = Search and Replace String(input string=w302, search string="/Value  **", replace string="/Direction") -> (result string=w308:string)  [unwired: 5 in, 3 out]
            n166 = property on="Test Ring" class="Ring (strict)"("Visible"=w301) -> ()  [unwired: 2 in, 2 out]
            n167 = call <vilib>:"NT Read String.vi"("Name"=w308) -> ("String"=w306:string)  [unwired: 9 in, 1 out]
            n168 = Equal?(x="Both directions", y=w306) -> (x = y?=w304:bool)
            n169 = Not(x=w304) -> (.not. x?=w305:bool)
            n170 = property on="Rev/Fwd" class="Clust (strict)"("Visible"=w304) -> ()  [unwired: 2 in, 2 out]
            n171 = property on="On/Off" class="Bool (strict)"("Visible"=w305, "Caption.Text"=w303) -> ()  [unwired: 2 in, 2 out]
          }
          frame "Compressor", "Digital Out" {
            w311 = FALSE ("Visible")
            # "Get direction and finish"
            n172 = property on="Motor" class="Clust (strict)"("Visible"=w311) -> ()  [unwired: 2 in, 2 out]
            n173 = property on="Test Slider" class="Slide (strict)"("Visible"=w311) -> ()  [unwired: 2 in, 2 out]
            n174 = property on="Test Ring" class="Ring (strict)"("Visible"=w311) -> ()  [unwired: 2 in, 2 out]
            n175 = property on="On/Off" class="Bool (strict)"("Visible"=TRUE, "Caption.Text"=w312) -> ()  [unwired: 2 in, 2 out]
            n176 = property on="Rev/Fwd" class="Clust (strict)"("Visible"=FALSE) -> ()  [unwired: 2 in, 2 out]
          }
          frame "Camera" {
            n177 = call <vilib>:"Get Last Path Segment.vi"("String in"=w319) -> ("String out"=w320:string)  [unwired: 10 in]
            n178 = property on="On/Off" class="Bool (strict)"("Visible"=FALSE) -> ()  [unwired: 2 in, 2 out]
            n179 = property on="Motor" class="Clust (strict)"("Visible"=FALSE) -> ()  [unwired: 2 in, 2 out]
            n180 = property on="Rev/Fwd" class="Clust (strict)"("Visible"=FALSE) -> ()  [unwired: 2 in, 2 out]
            n181 = case shown="\"White Balance  **\"" w320 {
              tunnel: w319 -> [w326 w335 w344 w353 w362 _ w368]
              tunnel: w318 -> [w324 w332 w341 w350 w359 _ _]
              frame "Size  **" {
                n182 = Index Array(array=w324) -> (element=w323:cluster{string[]})  [unwired: 1 in]
                n183 = call <vilib>:"NT Read String.vi"("Name"=w326) -> ("String"=w325:string)  [unwired: 9 in, 1 out]
                n184 = Unbundle(w323) -> (w321:string[])
                n185 = Match First String(2:w321, 3:w325) -> (0:w322:i32)  [unwired: 1 out]
                n186 = property on="Test Ring" class="Ring (strict)"("Value"=w322, "Strings []"=w321) -> ()  [unwired: 2 in, 2 out]
                n187 = property on="Test Ring" class="Ring (strict)"("Visible"=TRUE) -> ()  [unwired: 2 in, 2 out]
                n188 = property on="Test Slider" class="Slide (strict)"("Visible"=FALSE) -> ()  [unwired: 2 in, 2 out]
              }
              frame "White Balance  **" {
                n189 = Index Array(array=w332, index=1) -> (element=w333:cluster{string[]})
                n190 = call <vilib>:"NT Read String.vi"("Name"=w335) -> ("String"=w334:string)  [unwired: 9 in, 1 out]
                n191 = Unbundle(w333) -> (w330:string[])
                n192 = Match First String(2:w330, 3:w334) -> (0:w329:i32)  [unwired: 1 out]
                n193 = property on="Test Ring" class="Ring (strict)"("Value"=w329, "Strings []"=w330) -> ()  [unwired: 2 in, 2 out]
                n194 = property on="Test Ring" class="Ring (strict)"("Visible"=TRUE) -> ()  [unwired: 2 in, 2 out]
                n195 = property on="Test Slider" class="Slide (strict)"("Visible"=FALSE) -> ()  [unwired: 2 in, 2 out]
              }
              frame "Exposure  **" {
                n196 = Index Array(array=w341, index=2) -> (element=w342:cluster{string[]})
                n197 = call <vilib>:"NT Read String.vi"("Name"=w344) -> ("String"=w343:string)  [unwired: 9 in, 1 out]
                n198 = Unbundle(w342) -> (w338:string[])
                n199 = Match First String(2:w338, 3:w343) -> (0:w339:i32)  [unwired: 1 out]
                n200 = property on="Test Ring" class="Ring (strict)"("Value"=w339, "Strings []"=w338) -> ()  [unwired: 2 in, 2 out]
                n201 = property on="Test Ring" class="Ring (strict)"("Visible"=TRUE) -> ()  [unwired: 2 in, 2 out]
                n202 = property on="Test Slider" class="Slide (strict)"("Visible"=FALSE) -> ()  [unwired: 2 in, 2 out]
              }
              frame "Exposure Priority  **" {
                n203 = Index Array(array=w350, index=3) -> (element=w351:cluster{string[]})
                n204 = call <vilib>:"NT Read String.vi"("Name"=w353) -> ("String"=w352:string)  [unwired: 9 in, 1 out]
                n205 = Unbundle(w351) -> (w347:string[])
                n206 = Match First String(2:w347, 3:w352) -> (0:w348:i32)  [unwired: 1 out]
                n207 = property on="Test Ring" class="Ring (strict)"("Value"=w348, "Strings []"=w347) -> ()  [unwired: 2 in, 2 out]
                n208 = property on="Test Ring" class="Ring (strict)"("Visible"=TRUE) -> ()  [unwired: 2 in, 2 out]
                n209 = property on="Test Slider" class="Slide (strict)"("Visible"=FALSE) -> ()  [unwired: 2 in, 2 out]
              }
              frame "Color Enable  **" {
                n210 = Index Array(array=w359, index=4) -> (element=w360:cluster{string[]})
                n211 = call <vilib>:"NT Read String.vi"("Name"=w362) -> ("String"=w361:string)  [unwired: 9 in, 1 out]
                n212 = Unbundle(w360) -> (w356:string[])
                n213 = Match First String(2:w356, 3:w361) -> (0:w357:i32)  [unwired: 1 out]
                n214 = property on="Test Ring" class="Ring (strict)"("Value"=w357, "Strings []"=w356) -> ()  [unwired: 2 in, 2 out]
                n215 = property on="Test Ring" class="Ring (strict)"("Visible"=TRUE) -> ()  [unwired: 2 in, 2 out]
                n216 = property on="Test Slider" class="Slide (strict)"("Visible"=FALSE) -> ()  [unwired: 2 in, 2 out]
              }
              frame Default {
                n217 = property on="Test Ring" class="Ring (strict)"("Visible"=FALSE) -> ()  [unwired: 2 in, 2 out]
                n218 = property on="Test Slider" class="Slide (strict)"("Visible"=FALSE) -> ()  [unwired: 2 in, 2 out]
              }
              frame "Brightness  **", "Color Level  **", "Compression  **", "FPS  **", "Sharpness  **" {
                n219 = call <vilib>:"NT Read Number.vi"("Name"=w368) -> ("Numeric"=w367:dbl)  [unwired: 9 in, 1 out]
                n220 = local write "Test Slider"(w367) -> ()
                n221 = property on="Test Slider" class="Slide (strict)"("Visible"=TRUE, "Scale.Maximum"=100.0 ("Scale.Range:Maximum")) -> ()  [unwired: 2 in, 2 out]
                n222 = property on="Test Ring" class="Ring (strict)"("Visible"=FALSE) -> ()  [unwired: 2 in, 2 out]
              }
            }
          }
        }
        n223 = property on="Progress" class="Clust (strict)"("Visible"=FALSE) -> ()  [unwired: 2 in, 2 out]
      }
      event "Test Name": Mouse Enter {
        # "Populate the ring with the list of tests"
        n224 = event-data() -> ()  [unwired: 1 in, 1 out]
        n225 = call <vilib>:"NT Read String Array.vi"("Name"="TestMode/TestList") -> ("String Array"=w376:string[])  [unwired: 9 in, 1 out]
        n226 = Build Array (concatenate)("Select the test to run...", w376) -> (w375:string[])
        n227 = property on="Test Name" class="Ring (strict)"("Strings []"=w375) -> ()  [unwired: 2 in, 2 out]
      }
      event "Test Name": Value Change {
        w378 = FALSE ("Visible")
        # "Tell the robot the test name to run"
        n228 = event-data() -> ("NewVal"=w382:u16)  [unwired: 1 in]
        n229 = property on="Test Name" class="Ring (strict)"() -> ("Strings []"=w383:string[])  [unwired: 2 in, 2 out]
        n230 = local write "Progress"(T6 {"Test Progress"=0, "Test Progress Text"=""} ("Progress")) -> ()
        n231 = Index Array(array=w383, index=w382) -> (element=w381:string)
        n232 = call <vilib>:"NT Write String.vi"("String"=w381, "Name"="TestMode/TestName") -> ()  [unwired: 9 in, 1 out]
        n233 = property on="Progress" class="Clust (strict)"("Visible"=TRUE) -> ()  [unwired: 2 in, 2 out]
        n234 = property on="Motor" class="Clust (strict)"("Visible"=w378) -> ()  [unwired: 2 in, 2 out]
        n235 = property on="Test Slider" class="Slide (strict)"("Visible"=w378) -> ()  [unwired: 2 in, 2 out]
        n236 = property on="On/Off" class="Bool (strict)"("Visible"=w378) -> ()  [unwired: 2 in, 2 out]
        n237 = property on="Rev/Fwd" class="Clust (strict)"("Visible"=w378) -> ()  [unwired: 2 in, 2 out]
        n238 = property on="Test Ring" class="Ring (strict)"("Visible"=w378) -> ()  [unwired: 2 in, 2 out]
      }
      event "Select Auto": Mouse Enter {
        # "Populate the combo box with the list of autonomous options"
        n239 = event-data() -> ()  [unwired: 1 in, 1 out]
        n240 = call <vilib>:"NT Read String Array.vi"("Name"="Auto List") -> ("String Array"=w385:string[])  [unwired: 9 in, 1 out]
        n241 = property on="Select Auto" class="CmbBox"("Strings[]"=w385) -> ()  [unwired: 2 in, 2 out]
      }
      event "Select Auto": Value Change {
        # "User modified the Auto Selection. Write to NT variable so robot knows."
        n242 = event-data() -> ("NewVal"=w388:string)  [unwired: 1 in]
        n243 = call <vilib>:"NT Write String.vi"("String"=w388, "Name"="Auto Selector") -> ()  [unwired: 9 in, 1 out]
      }
      event "Command Selection": Value Change {
        # "Get the params and show in table"
        n244 = event-data() -> ("NewVal"=w394:i32)  [unwired: 1 in]
        n245 = property on="Command Selection" class="MCListbox (strict)"() -> ("ItemNames"=w392:string[][])  [unwired: 2 in, 2 out]
        n246 = call <vilib>:"WPI_DashboardUpdate Command Params.vi"("NewVal"=w394, "Commands"=w392, "Param Tbl"=w393) -> ()  [unwired: 8 in, 1 out]
      }
      event "Execute Command": Value Change {
        # "Started one, Unique ID holds\nresponse"
        n247 = event-data() -> ()  [unwired: 1 in, 1 out]
        n248 = property on="Command Selection" class="MCListbox (strict)"() -> ("ItemNames"=w405:string[][])  [unwired: 2 in, 2 out]
        n249 = Index Array(array=w405, index (row)="Command Selection", index (col)=0) -> (element=w403:string)
        n250 = call <vilib>:"Invoke Commands.vi"("Command Params"="Command Params", "Function Name"=w403) -> ("Params"=w399:u8, "Started"=w398:bool)  [unwired: 7 in, 1 out]
        n251 = Array Subset(array="Command Params", length (row)=w399) -> (w400:string[][])  [unwired: 3 in]
        n252 = Select(t="Executing" ("Cmd Status"), s=w398, f="" ("Cmd Status")) -> (s? t:f=→"Cmd Status":string)
      }
      event "Command Selection": Double Click {
        n253 = event-data() -> ("Row"=w413:i32)  [unwired: 1 in]
        n254 = property on="Command Selection" class="MCListbox (strict)"() -> ("ItemNames"=w416:string[][])  [unwired: 2 in, 2 out]
        n255 = local read "Command Params"() -> (w412:string[][])
        n256 = Index Array(array=w416, index (row)=w413, index (col)=0) -> (element=w414:string)
        n257 = call <vilib>:"Invoke Commands.vi"("Command Params"=w412, "Function Name"=w414) -> ("Params"=w411:u8, "Started"=w406:bool)  [unwired: 7 in, 1 out]
        n258 = Array Subset(array=w412, length (row)=w411) -> (w410:string[][])  [unwired: 3 in]
        n259 = Select(t="Executing" ("Cmd Status"), s=w406, f="" ("Cmd Status")) -> (s? t:f=w407:string)
        n260 = local write "Cmd Status"(w407) -> ()
      }
      event "CheckList": Double Click {
        # "Shift clears all"
        # "Update symbols on the listbox"
        n261 = event-data() -> ("PlatMods.Shift"=w418:bool, "Row"=w420:i32)  [unwired: 1 in]
        n262 = case shown="True" w418 {
          tunnel: w420 -> [w424 _]
          tunnel: 1 -> [w423 _]
          frame False {
            n263 = property on="CheckList" class="LstBox (strict)"() -> ("Item Symbols"=w422:i32[])  [unwired: 2 in, 2 out]
            n264 = Replace Array Subset(array=w422, new element=w423, index=w424) -> (w421:i32[])
            n265 = property on="CheckList" class="LstBox (strict)"("Item Symbols"=w421) -> ()  [unwired: 2 in, 2 out]
          }
          frame True {
            w425 = 0 ("Top Row")
            n266 = property on="CheckList" class="LstBox (strict)"() -> ("Number of Rows"=w427:u32)  [unwired: 2 in, 2 out]
            n267 = Initialize Array(0, w427) -> (w426:i32[])
            n268 = property on="CheckList" class="LstBox (strict)"("Top Row"=w425, "Value"=w425, "Item Symbols"=w426) -> ()  [unwired: 2 in, 2 out]
          }
        }
      }
      event "CheckList": Key Down {
        # "Update symbols on the listbox\nLeft and right keys check and uncheck"
        n269 = event-data() -> ("VKey"=w431:T23)  [unwired: 1 in]
        n270 = case shown="\"Left\", \"Right\"" w431 {
          selector: w431 -> [w436 _]
          tunnel: eventvkey."Left" ("VKey") -> [w434 _]
          frame "Left", "Right" {
            n271 = Equal?(x=w434, y=w436) -> (x = y?=w435:bool)
            n272 = Select(t=0, s=w435, f=1) -> (s? t:f=w437:i32)
            n273 = property on="CheckList" class="LstBox (strict)"() -> ("Item Symbols"=w440:i32[])  [unwired: 2 in, 2 out]
            n274 = Replace Array Subset(array=w440, new element=w437, index="CheckList") -> (w439:i32[])
            n275 = property on="CheckList" class="LstBox (strict)"("Item Symbols"=w439) -> ()  [unwired: 2 in, 2 out]
          }
          frame Default {
          }
        }
      }
      event "Motor.Enable": Value Change {
        # "When the test mode otor enable helper is set, update that\ntree row item's value"
        n276 = event-data() -> ("NewVal"=w446:bool)  [unwired: 1 in]
        n277 = Unbundle("Motor") -> ("Value"=w445:dbl)  [unwired: 1 out]
        n278 = Select(t=w445, s=w446, f=0.0) -> (s? t:f=w443:dbl)
        n279 = call <vilib>:"NT Write Number.vi"("Numeric"=w443, "Name"=w442) -> ()  [unwired: 9 in, 1 out]
      }
      event "Test Slider": Value Change {
        # "When the test mode slider helper is set, update that\ntree row item's value"
        n280 = event-data() -> ("NewVal"=w449:dbl)  [unwired: 1 in]
        n281 = call <vilib>:"NT Write Number.vi"("Numeric"=w449, "Name"=w450) -> ()  [unwired: 9 in, 1 out]
      }
      event "On/Off": Value Change {
        # "When the test mode on/off helper value is set, update that\ntree row item's value"
        n282 = event-data() -> ("NewVal"=w454:bool)  [unwired: 1 in]
        n283 = Boolean To (0,1)(Boolean=w454) -> (0, 1=w453:i16)
        n284 = call <vilib>:"NT Write Number.vi"("Numeric"=w453, "Name"=w452) -> ()  [unwired: 9 in, 1 out]
      }
      event "Rev/Fwd": Value Change {
        # "When the test mode helper value for relays is set, update that\ntree row item's value"
        n285 = event-data() -> ("NewVal.Forward"=w462:bool, "NewVal.Reverse"=w461:bool)  [unwired: 1 in]
        n286 = Boolean To (0,1)(Boolean=w462) -> (0, 1=w458:i16)
        n287 = Boolean To (0,1)(Boolean=w461) -> (0, 1=w460:i16)
        n288 = Negate(x=w460) -> (-x=w459:i16)
        n289 = Add(x=w458, y=w459) -> (x+y=w457:i16)
        n290 = call <vilib>:"NT Write Number.vi"("Numeric"=w457, "Name"=w456) -> ()  [unwired: 9 in, 1 out]
      }
      event "Test Ring": Value Change {
        # "When a test mode helper value is selected from the ring,\nset the tree item's variable to the string value"
        n291 = event-data() -> ("NewVal"=w466:u16)  [unwired: 1 in]
        n292 = property on="Test Ring" class="Ring (strict)"() -> ("Strings []"=w467:string[])  [unwired: 2 in, 2 out]
        n293 = Index Array(array=w467, index=w466) -> (element=w465:string)
        n294 = call <vilib>:"NT Write String.vi"("String"=w465, "Name"=w464) -> ()  [unwired: 9 in, 1 out]
      }
      event "Rec Mode": Value Change {
        # "Update globals for recording mode and path to read log from.\nClear when logging and let NetworkTables set path for vision to\nuse."
        n295 = event-data() -> ("NewVal"=w478:enum32{"Stop", "Record", "Playback"})  [unwired: 1 in]
        n296 = global write "WPI_DashboardLogging Global.vi" "Logging Filename"(path "") -> ()
        n297 = global write "WPI_DashboardLogging Global.vi" "Recording"(w478) -> ()
        n298 = case shown="\"Playback\"" w478 {
          tunnel: w477 -> [_ w480 w489]
          tunnel: [_ _ w488] -> w475
          tunnel: [_ _ w487] -> _
          tunnel: w473 -> [_ _ w485]
          tunnel: cluster{i32, i32} {-250, 170} -> [_ _ w484]
          tunnel: [_ _ T24 {"Image Size"=TRUE, "Image Type"=TRUE, "Pixel Value"=TRUE, "ROI Information"=TRUE, "Zoom Factor"=FALSE} ("Image Information Shown:All Elements")] -> w468
          tunnel: [_ _ TRUE ("Zoom Factor")] -> w469
          tunnel: w471 -> [_ _ w481]
          frame Default {
          }
          frame "Stop", "Record" {
            # "Place Window too"
            n299 = invoke class="VI" method="FP.Close"(reference=w480) -> (reference out=w479:refnum<vi>)  [unwired: 2 in, 2 out]
            n300 = invoke class="VI" method="Abort VI"(reference=w479) -> ()  [unwired: 2 in, 3 out]
          }
          frame "Playback" {
            n301 = call "Open Playback Panel.vi"("Offset"=w484, "DB VI Ref"=w485, "Playback in"=w489) -> ("Playback out"=w486:refnum<vi>)  [unwired: 8 in]
            n302 = register-events(w486, w481) -> (reference out=w488:refnum<event-registration>, error out=w487:errorcluster)  [unwired: 2 in]
          }
        }
        n303 = property on="Camera Image Right" class="ImageControl"("Image Information Shown"=w468, "Image Information Visible"=w469) -> ()  [unwired: 2 in, 2 out]
        n304 = property on="Camera Image" class="ImageControl"("Image Information Shown"=w468, "Image Information Visible"=w469) -> ()  [unwired: 2 in, 2 out]
        n305 = call <vilib>:"WPI_DashboardNT Log FieldName Cache.vi"("Operation"=enum16{"Lookup/Add", "Index", "Clear"}."Clear") -> ()  [unwired: 8 in, 3 out]
      }
      event Panel Close {
        w491 = enum32{"Stop", "Record", "Playback"}."Stop" ("Rec Mode")
        # "Playback window has been closed, abort"
        n306 = event-data() -> ()  [unwired: 1 in, 4 out]
        n307 = local write "Rec Mode"(w491) -> ()
        n308 = global write "WPI_DashboardLogging Global.vi" "Recording"(w491) -> ()
      }
      event Panel Close {
        # "Abort playback window and ourself"
        n309 = event-data() -> ()  [unwired: 1 in, 4 out]
        n310 = invoke class="VI" method="FP.Close"(reference=w495) -> (reference out=w494:refnum<vi>)  [unwired: 2 in, 2 out]
        n311 = invoke class="VI" method="Abort VI"(reference=w494) -> (error out=w493:errorcluster)  [unwired: 2 in, 2 out]
        n312 = invoke class="VI" method="Abort VI"(error in=w493) -> ()  [unwired: 2 in, 3 out]
      }
      event User Event {
        n313 = event-data() -> ("IDs"=w502:cluster{"RPC field ID":u16, "Unique ID":u16}, "String"=w501:string)  [unwired: 1 in]
        n314 = Bundle("IDs"=w502, "String"=w501) -> (w500:T10)  [unwired: 1 in]
        n315 = call <vilib>:"Retrieve RPC Response.vi"("RPC Response"=w500) -> ("Output"=w498:string[][])  [unwired: 10 in]
        n316 = Build Array (concatenate)(w496, w498) -> (w497:string[][])
        n317 = local write "Command Params"(w497) -> ()
        n318 = local write "Cmd Status"("" ("Cmd Status")) -> ()
      }
      event "Tree": Double Click {
        n319 = event-data() -> ("PlatMods"=w508:T27, "Tag"=w505:string)  [unwired: 1 in]
        n320 = Unbundle(w508) -> ("Shift"=w507:bool)  [unwired: 4 out]
        n321 = String Subset(string=w505, length (rest)=1 ("length (rest)")) -> (substring=w504:string)  [unwired: 1 in]
        n322 = Not(x=w507) -> (.not. x?=w506:bool)
        n323 = case shown="\"/\"" w504 {
          tunnel: w505 -> [_ w511]
          tunnel: w506 -> [_ w510]
          frame Default {
          }
          frame "/" {
            n324 = call <vilib>:"NT Update Persistence.vi"("Persistence"=w510, "Name"=w511) -> ()  [unwired: 9 in, 1 out]
          }
        }
      }
    }
  }
  n325 = while {
    tunnel: w65 -> [w513]
    i -> [w516]
    stop <- FALSE stop-if-true
    n326 = Wait (ms)(milliseconds to wait=u32 100) -> ()  [unwired: 1 out]
    n327 = case shown="\"Playback\"" "Rec Mode" {
      tunnel: w516 -> [_ _ w531]
      tunnel: [u32 2829099 ("Base Color") u32 11141120 ("Target Color") w520] -> w512
      frame "Stop", Default {
        # "Reset the color, extra updates don't cost much"
      }
      frame "Record" {
      }
      frame "Playback" {
        # "Playback"
        n328 = Quotient & Remainder(x=w531, y=u32 50 ("milliseconds to wait")) -> (x-y*floor(x/y)=w527:u32)  [unwired: 1 out]
        n329 = Divide(x=w527, y=u32 50 ("milliseconds to wait")) -> (x/y=w524:dbl)
        n330 = Multiply(x=6.283185307179586, y=w524) -> (x*y=w529:dbl)
        n331 = Sine(x=w529) -> (sin(x)=w528:dbl)
        n332 = Absolute Value(x=w528) -> (abs(x)=w521:dbl)
        n333 = call "Interpolate RGB Color.vi"("Proportion"=w521, "Target Color"=u32 30976, "Base Color"=u32 2829099) -> ("Result Color"=w520:u32)  [unwired: 8 in]
      }
    }
    n334 = property class="Pane"(reference=w513, "PaneColor"=w512) -> ()  [unwired: 1 in, 2 out]
  }
  n335 = local write "Dashboard Tab"(T2."Drive" ("Dashboard Tab")) -> ()
  n336 = property on="On/Off" class="Bool (strict)"("Visible"=w36) -> ()  [unwired: 2 in, 2 out]
  n337 = property on="Motor" class="Clust (strict)"("Visible"=w36) -> ()  [unwired: 2 in, 2 out]
  n338 = property on="Progress" class="Clust (strict)"("Visible"=w36) -> ()  [unwired: 2 in, 2 out]
  n339 = property on="Test Ring" class="Ring (strict)"("Visible"=w36) -> ()  [unwired: 2 in, 2 out]
  n340 = property on="Rev/Fwd" class="Clust (strict)"("Visible"=w36) -> ()  [unwired: 2 in, 2 out]
  n341 = while {
    tunnel: u16 1741 ("timeout ms (25000)") -> [w533]
    stop <- FALSE stop-if-true
    n342 = TCP Create Listener(10:w533) -> (0:w532:errorcluster, 3:w534:refnum<k5>)  [unwired: 4 in, 1 out]
    n343 = case shown="No Error" w532 {
      selector: w532 -> [w536 _]
      tunnel: w534 -> [w537 _]
      frame No Error {
        n344 = while {
          tunnel: w537 -> [w540]
          tunnel: w536 -> [w539]
          stop <- FALSE stop-if-true
          n345 = TCP Wait On Listener(8:w539, 11:w540) -> (0:w541:errorcluster, 4:w542:refnum<k5>)  [unwired: 2 in, 3 out]
          n346 = local write "TCP"(w542) -> ()
          n347 = case shown="No Error" w541 {
            frame No Error {
            }
            frame Error {
              n348 = Wait (ms)(milliseconds to wait=u32 1000) -> ()  [unwired: 1 out]
            }
          }
        }
      }
      frame Error {
        n349 = Wait (ms)(milliseconds to wait=u32 1000) -> ()  [unwired: 1 out]
      }
    }
  }
  n350 = local write "Command Selection"(u16 0 ("milliseconds to wait")) -> ()
  n351 = local write "Command Params"(string[][] [] ("Command Params")) -> ()
  n352 = global write "WPI_DashboardLogging Global.vi" "Recording"(w59) -> ()
  n353 = local write "Rec Mode"(w59) -> ()
  n354 = call <vilib>:"NT Write String.vi"("String"="Select Auto", "Name"="Auto Selector") -> ()  [unwired: 9 in, 1 out]
